vi "Init shared library.vi"(8 "error in (no error)":errorcluster) -> (0 "error out":errorcluster)   [LabVIEW 2017]
uses:
  Variables/MyRIO Lidar Class Data.vi
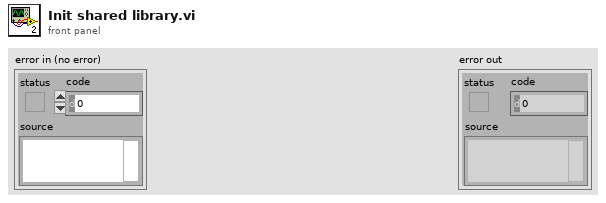
[diagram p1: front panel]
types:
  T1 = cluster{"Shared library path":path, "File Descriptor":i32}
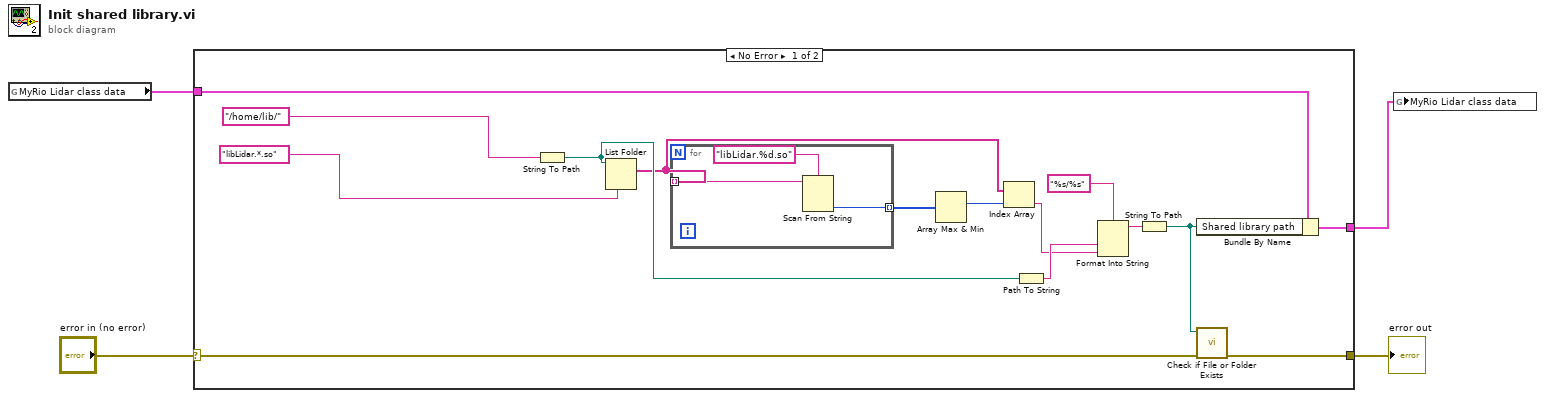
[diagram p0: block diagram]
diagram:
  n1 = global read "MyRIO Lidar Class Data.vi" "MyRio Lidar class data"() -> (w2:T1)
  n2 = case shown="No Error" "error in (no error)" {
    selector: "error in (no error)" -> [w9 w24]
    tunnel: [w8 w24] -> w3
    tunnel: w2 -> [w6 w23]
    tunnel: [w5 w23] -> w1
    frame No Error {
      n3 = String To Path(string="/home/lib/") -> (path=w19:path)
      n4 = List Folder(path=w19, pattern="libLidar.*.so") -> (filenames=w13:string[])  [unwired: 2 in, 3 out]
      n5 = for {
        tunnel: w13 -> [w22] mode=indexing
        tunnel: [w20] -> w12 mode=indexing
        n6 = Scan From String(format string="libLidar.%d.so", input string=w22) -> (output 1=w20:i32)  [unwired: 3 in, 3 out]
      }
      n7 = Array Max & Min(array=w12) -> (max index (indices)=w14:i32)  [unwired: 3 out]
      n8 = Index Array(array=w13, index=w14) -> (element=w16:string)
      n9 = Path To String(path=w19) -> (string=w17:string)
      n10 = Format Into String(format string="%s/%s", w17, w16) -> (resulting string=w18:string)  [unwired: 2 in, 1 out]
      n11 = String To Path(string=w18) -> (path=w7:path)
      n12 = Bundle By Name(cluster=w6, "Shared library path"=w7) -> (w5:T1)
      n13 = call <vilib>:"Check if File or Folder Exists.vi"("error in (no error)"=w9, "path"=w7) -> ("error out"=w8:errorcluster)  [unwired: 7 in, 2 out]
    }
    frame Error {
    }
  }
  "error out" <- w3
  n14 = global write "MyRIO Lidar Class Data.vi" "MyRio Lidar class data"(w1) -> ()
